vi "Output_true_Sub.vi"(1 "Write to terminal":bool) -> (0 "Boolean":bool)   [LabVIEW 2010]
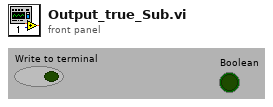
[diagram p1: front panel]
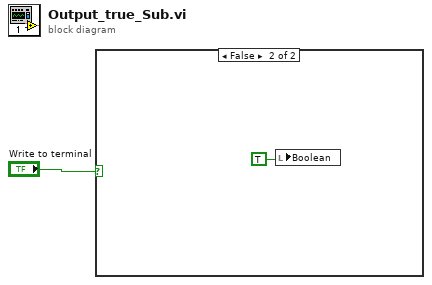
[diagram p0: block diagram]
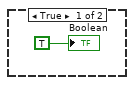
[diagram p2: hidden frame]
diagram:
  n1 = case shown="False" "Write to terminal" {
    frame True {
      "Boolean" <- TRUE ("Boolean")
    }
    frame False {
      n2 = local write "Boolean"(TRUE ("Boolean")) -> ()
    }
  }
